vi "_Request Malloc MDPtrQ To Factory.vi"(10 "error in (no error)":errorcluster) -> (2 "error out":errorcluster, 3 "MDPtrQueue":T1)   [LabVIEW 2017, in "MDPtr.lvlib" / "MDPtrMgr.lvclass"]
uses:
  MDPtrMgr.lvclass
  MDPtr TypeDef/MDPtr Queue.ctl
  MDPtr TypeDef/MDPtr DataFrame-Memory.ctl
  MDPtr TypeDef/MDPtr DataFrame-Common.ctl
  <vilib>/Utility/Data Type/Type Definitions/Data Type.ctl
  Def-Request.ctl
  Def-Respone.ctl
  <vilib>/Utility/Data Type/NI_Data Type.lvlib
  MDPtr.lvlib
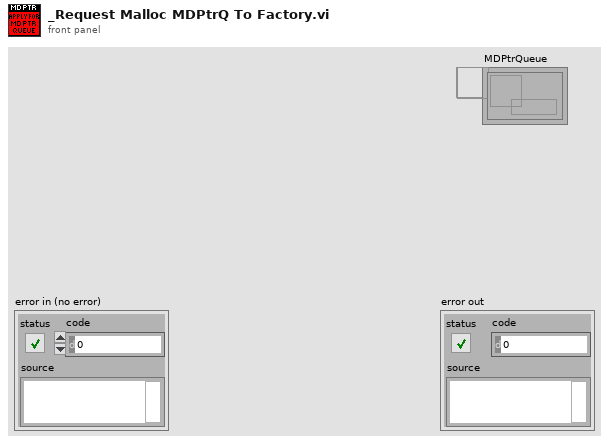
[diagram p1: front panel]
types:
  T1 = typedef "MDPtr.lvlib/MDPtr Queue.ctl" = refnum<queue>
  T2 = typedef "MDPtr.lvlib/MDPtrMgr.lvclass/Def-Respone.ctl" = cluster{"MDPtr DVR":refnum<data-value>, "error out":errorcluster, "MDPtrQueue":T1}
  T3 = typedef "MDPtr.lvlib/MDPtrMgr.lvclass/Def-Request.ctl" = cluster{"Type":enum16{"DVR", "Queue"}, "Cache Length":i32, "ResponeQueue":refnum<queue>}
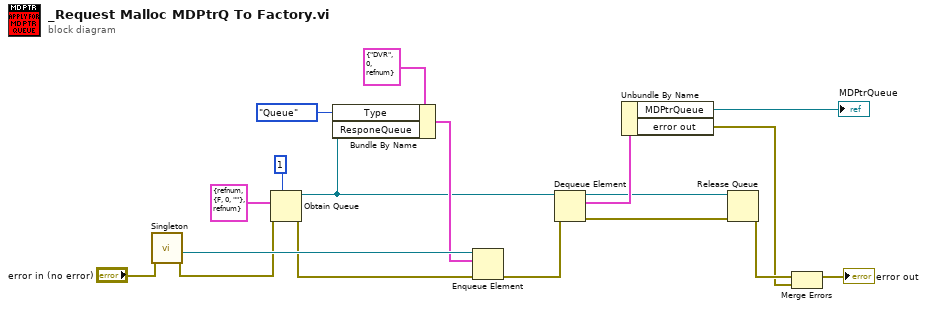
[diagram p0: block diagram]
diagram:
  n1 = call "Singleton.vi"("error in (no error)"="error in (no error)") -> ("error out"=w12:errorcluster, "RequestQueue"=w18:refnum<queue>)  [unwired: 8 in, 1 out]
  n2 = Obtain Queue(max queue size (-1, unlimited)=1, element data type=T2 {"MDPtr DVR"=refnum, "error out"={"status"=FALSE, "code"=0, "source"=""}, "MDPtrQueue"=refnum} ("Request"), error in (no error)=w12) -> (queue out=w9:refnum<queue>, error out=w11:errorcluster)  [unwired: 2 in, 1 out]
  n3 = Bundle By Name(cluster=T3 {"Type"=enum."DVR", "Cache Length"=0, "ResponeQueue"=refnum} ("element"), "Type"=enum16{"DVR", "Queue"}."Queue", "ResponeQueue"=w9) -> (w16:T3)
  n4 = Enqueue Element(queue=w18, element=w16, error in (no error)=w11) -> (error out=w8:errorcluster)  [unwired: 1 in, 2 out]
  n5 = Dequeue Element(queue=w9, error in (no error)=w8) -> (queue out=w6:refnum<queue>, element=w7:T2, error out=w5:errorcluster)  [unwired: 1 in, 1 out]
  n6 = Unbundle By Name(w7) -> ("MDPtrQueue"=→"MDPtrQueue":T1, "error out"=w2:errorcluster)
  n7 = Release Queue(queue=w6, error in (no error)=w5) -> (error out=w4:errorcluster)  [unwired: 1 in, 2 out]
  n8 = Merge Errors(w4, w2) -> (→"error out":errorcluster)
